vi "SMO.InstrumentDriver.GetPrivateEvents.vi"(8 "error in (no error)":errorcluster, 11 "SMO.InstrumentDriver":refnum<class "SMO.InstrumentDriver.lvclass">) -> (0 "error out":errorcluster, 2 "Private Events":T1, 3 "SMO.InstrumentDriver out":refnum<class "SMO.InstrumentDriver.lvclass">)   [LabVIEW 2013, in "SMO.InstrumentDriver.lvclass"]
doc: "---------------------------------------------------------------\nJKI State Machine Objects™\nhttp://jki.net/state-machine-objects/\nCopyright (C) 2005-2015, JKI <info@jki.net>\nALL RIGHTS RESERVEDJKI State Machine Objects (SMO) 1.0.0.4\nJKI - JKI\nCopyright (c) 2015, JKI"
uses:
  SMO.InstrumentDriver.lvclass
  Typedefs/PrivateEvents--Cluster.ctl
  Typedefs/WriteData.ctl
  SMO.InstrumentDriver.lvclass/SMO.InstrumentDriver.ctl
panel:
  # "For instructions on how to use the JKI State Machine Objects, examples and video tutorials, visit:\nhttp://jki.net/state-machine-objects/\n\nJKI State Machine Objects™\nhttp://jki.net/state-machine-objects/\nCopyright (C) 2005-2015, JKI <info@jki.net>\nALL RIGHTS RESERVED"
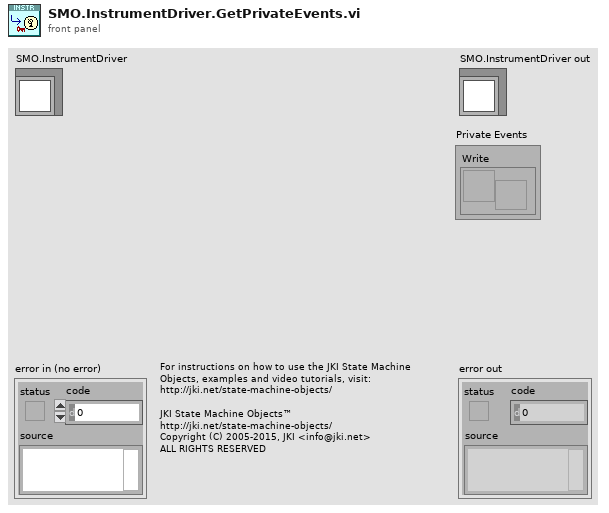
[diagram p1: front panel]
types:
  T1 = typedef "SMO.InstrumentDriver.lvclass/PrivateEvents--Cluster.ctl" = cluster{"Write":refnum<user-event>}
  T2 = typedef "SMO.InstrumentDriver.lvclass/PrivateData--Ref.ctl" = refnum<data-value>
  T3 = typedef "SMO.InstrumentDriver.lvclass/PrivateData--Cluster.ctl" = cluster{"Public Events":T4, "Private Events":T1}
  T4 = typedef "SMO.InstrumentDriver.lvclass/PublicEvents--Cluster.ctl" = cluster{"Value Changed":refnum<user-event>}
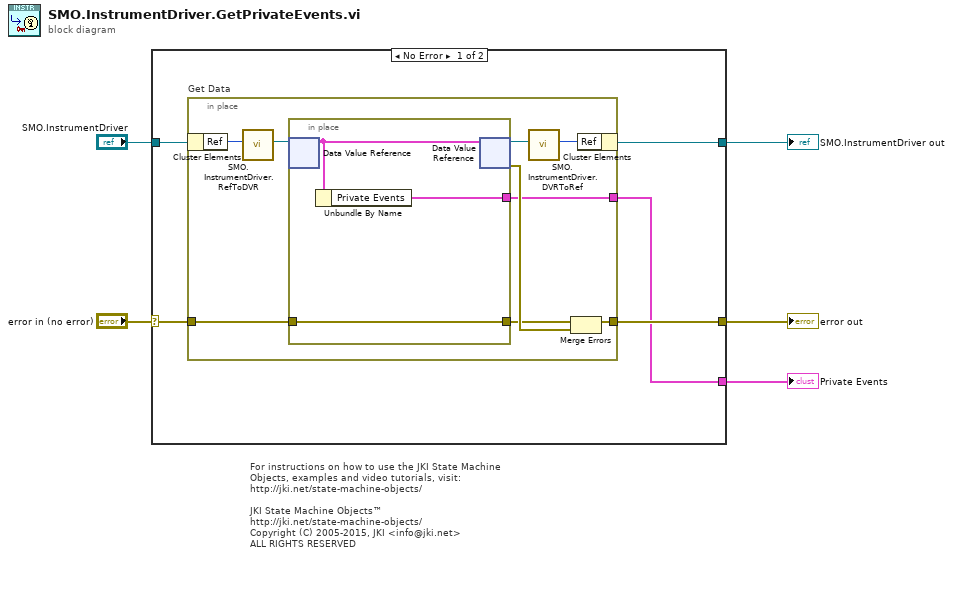
[diagram p0: block diagram]
diagram:
  # "For instructions on how to use the JKI State Machine Objects, examples and video tutorials, visit:\nhttp://jki.net/state-machine-objects/\n\nJKI State Machine Objects™\nhttp://jki.net/state-machine-objects/\nCopyright (C) 2005-2015, JKI <info@jki.net>\nALL RIGHTS RESERVED"
  n1 = case shown="No Error" "error in (no error)" {
    selector: "error in (no error)" -> [w9 w23]
    tunnel: "SMO.InstrumentDriver" -> [w10 w24]
    tunnel: [w7 w23] -> w4
    tunnel: [w8 w24] -> w3
    tunnel: [w6 _] -> w1
    frame No Error {
      n2 = in-place "Get Data" {
        in-place-border: w9 -> [w19]
        in-place-border: [w16] -> w7
        in-place-border: [w15] -> w6
        n3 = in-place-cluster #1(w10) -> ("Ref"=w14:u32)
        n4 = call "SMO.InstrumentDriver.RefToDVR.vi"("Ref"=w14) -> ("Ref"=w12:T2)  [unwired: 10 in]
        n5 = in-place {
          in-place-border: w19 -> [w21]
          in-place-border: [w21] -> w17
          in-place-border: [w20] -> w15
          n6 = in-place-dvr #2(w12) -> (w22:T3)  [unwired: 1 out]
          n7 = Unbundle By Name(w22) -> ("Private Events"=w20:T1)
          n8 = in-place-dvr #2(w22) -> (w13:T2, w18:errorcluster)
        }
        n9 = call "SMO.InstrumentDriver.DVRToRef.vi"("Ref"=w13) -> ("Ref"=w11:u32)  [unwired: 10 in]
        n10 = Merge Errors(w17, w18) -> (w16:errorcluster)
        n11 = in-place-cluster #1("Ref"=w11) -> (w8:refnum<class "SMO.InstrumentDriver.lvclass">)
      }
    }
    frame Error {
    }
  }
  "error out" <- w4
  "SMO.InstrumentDriver out" <- w3
  "Private Events" <- w1
